vi "Read_I64.vi"(8 "error in (no error)":errorcluster, 9 "offset":i32, 11 "tag handle":i32) -> (0 "error out":errorcluster, 2 "tag value":i64, 3 "tag handle out":i32)   [LabVIEW 2019]
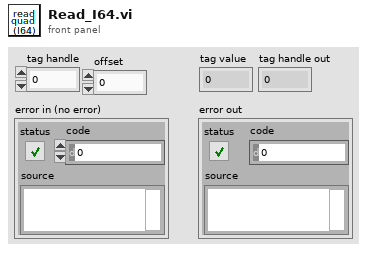
[diagram p1: front panel]
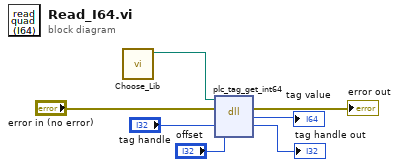
[diagram p0: block diagram]
diagram:
  n1 = call "Choose_Lib.vi"() -> ("appended path"=w1:path)  [unwired: 11 in]
  n2 = dll-call lib="home/dbowden/Desktop/libplctag-master/build/bin_dist/libplctag.so" fn="plc_tag_get_int64"(path in=w1, error in="error in (no error)", "tag"="tag handle", "offset"="offset") -> (error out=→"error out":errorcluster, "return type"=→"tag value":i64, "tag"=→"tag handle out":i32)  [unwired: 2 in, 1 out]
